vi "uTTA_CutCoolingToSection.vi"(4 "uTTA_MetaData":T1={"Tsamp,fast"=1.25, "Tsamp,slow"=20480.0, "Samples/Decade"=200, "Max.Divider"=14, "T_Preheat"=60.0, "T_Heat"=2400.0, "T_Cool"=10800.0, "Cooling Start Block"=601, " Total Blocks"=3250, "SuspectLines"=[], "Cool Voltage"=0.0, "Cool Volt Deviation"=0.0, "Heating Power"=0.0, "Chip Size"=0.0, "Interpolation Offset"=0.0, "Interpolation Factor m"=0.0, "No Suspect Lines"=0} {"No Suspect Lines" format="%.3pV"; "Interpolation Factor m" format="%.2g"; "Interpolation Offset" format="%.2g"; "Chip Size" format="%.2gmm²"; "Heating Power" format="%.3pW"; "Cool Volt Deviation" format="%.3pV"; "Cool Voltage" format="%.3pV"}, 5 "MeasData_in":T2, 6 "Off-Voltage":dbl=0.3 caption="Treshhold" min=-10.0 max=10.0 step=0.01, 7 "Cut at Off-Voltage":bool=TRUE caption="Enable") -> (0 "uTTA_MetaData_out":T1 {"No Suspect Lines" format="%.3pV"; "Interpolation Factor m" format="%.2g"; "Interpolation Offset" format="%.2g"; "Chip Size" format="%.2gmm²"; "Heating Power" format="%.3pW"; "Cool Volt Deviation" format="%.3pV"; "Cool Voltage" format="%.3pV"; "Tsamp,fast" format="%#_3gus"; "Tsamp,slow" format="%#_3gus"; "T_Preheat" format="%#_3gs"; "T_Heat" format="%#_3gs"; "T_Cool" format="%#_3gs"}, 1 "MeasData_out":T2, 2 "Index":i32, 3 "Graph_out":cluster{"Array":dbl[], "Array":dbl[]}[](array[cluster]))   [LabVIEW 2021]
uses:
  CTL_uTTA_MeasurementData.ctl
  uTTA_MetaData.ctl
  <vilib>/Analysis/NI_AALBase.lvlib
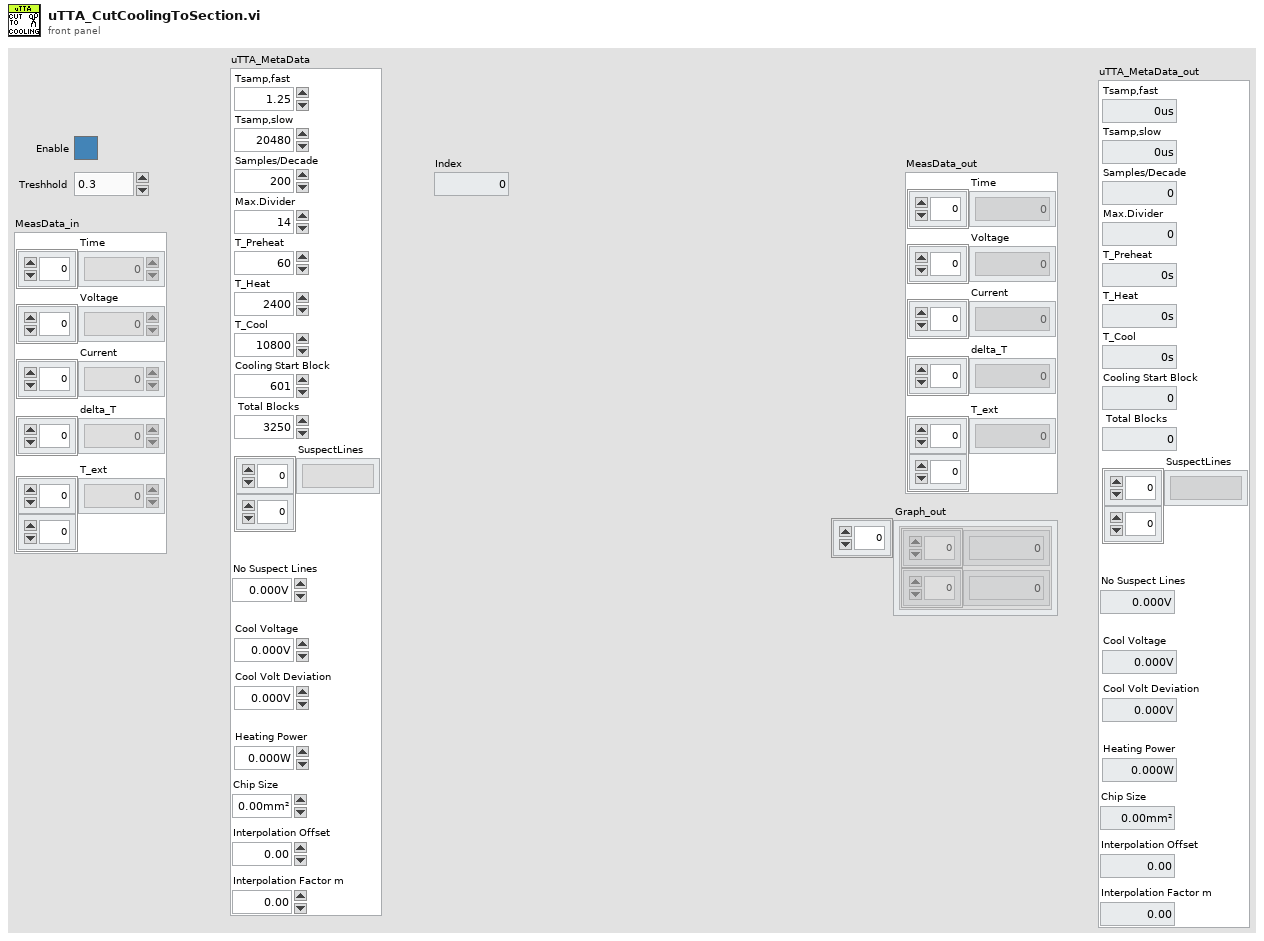
[diagram p1: front panel]
types:
  T1 = typedef "uTTA_MetaData.ctl" = cluster{"Tsamp,fast":dbl, "Tsamp,slow":dbl, "Samples/Decade":u32, "Max.Divider":u32, "T_Preheat":dbl, "T_Heat":dbl, "T_Cool":dbl, "Cooling Start Block":u32, " Total Blocks":u32, "SuspectLines":string[][], "Cool Voltage":dbl, "Cool Volt Deviation":dbl, "Heating Power":dbl, "Chip Size":dbl, "Interpolation Offset":dbl, "Interpolation Factor m":dbl, "No Suspect Lines":u32}
  T2 = typedef "CTL_uTTA_MeasurementData.ctl" = cluster{"Time":dbl[], "Voltage":dbl[], "Current":dbl[], "delta_T":dbl[], "T_ext":dbl[][]}
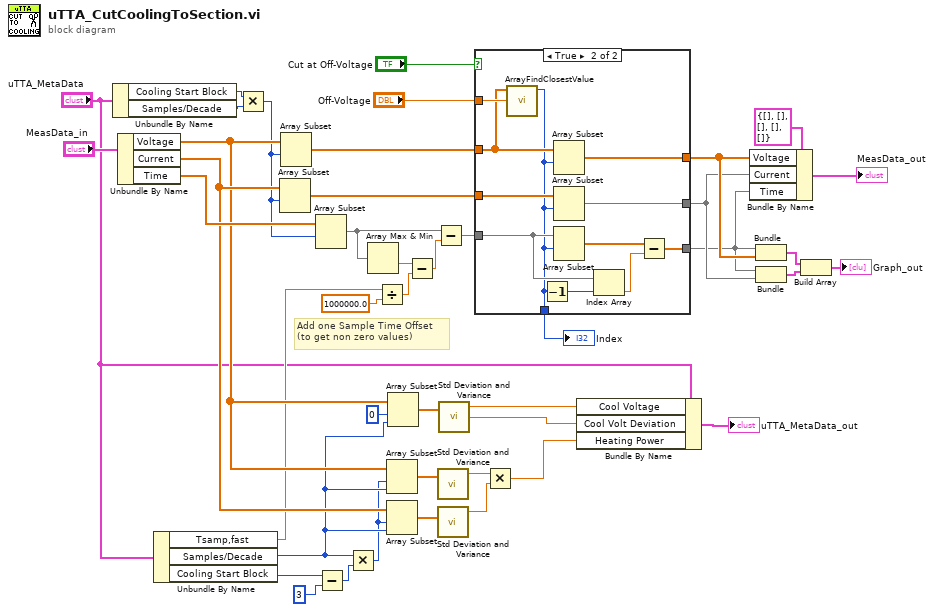
[diagram p0: block diagram]
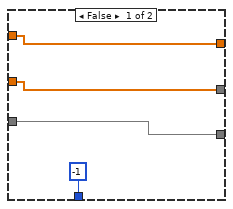
[diagram p2: hidden frame]
diagram:
  # "Add one Sample Time Offset\n(to get non zero values)"
  n1 = Unbundle By Name("uTTA_MetaData") -> ("Cooling Start Block"=w30:u32, "Samples/Decade"=w31:u32)
  n2 = Unbundle By Name("MeasData_in") -> ("Voltage"=w36:dbl[], "Current"=w37:dbl[], "Time"=w38:dbl[])
  n3 = Unbundle By Name("uTTA_MetaData") -> ("Tsamp,fast"=w34:dbl, "Samples/Decade"=w33:u32, "Cooling Start Block"=w32:u32)
  n4 = Multiply(x=w30, y=w31) -> (x*y=w14:u32)
  n5 = Array Subset(array=w37, index=w14) -> (w19:dbl[])  [unwired: 1 in]
  n6 = Array Subset(array=w36, index=w14) -> (w18:dbl[])  [unwired: 1 in]
  n7 = Array Subset(array=w38, index=w14) -> (w17:dbl[])  [unwired: 1 in]
  n8 = Subtract(x=w32, y=u32 3) -> (x-y=w24:u32)
  n9 = Multiply(x=w33, y=w24) -> (x*y=w25:u32)
  n10 = Array Max & Min(array=w17) -> (min value=w15:dbl)  [unwired: 3 out]
  n11 = Divide(x=w34, y=1000000.0) -> (x/y=w11:dbl)
  n12 = Array Subset(array=w36, index=w25, length=w33) -> (w26:dbl[])
  n13 = Array Subset(array=w37, index=w25, length=w33) -> (w27:dbl[])
  n14 = Array Subset(array=w36, index=0, length=w33) -> (w22:dbl[])
  n15 = Subtract(x=w15, y=w11) -> (x-y=w16:dbl)
  n16 = Subtract(x=w17, y=w16) -> (x-y=w20:dbl[])
  n17 = call <vilib>:"Std Deviation and Variance.vi"("X"=w26) -> ("mean"=w28:dbl)  [unwired: 1 in, 2 out]
  n18 = call <vilib>:"Std Deviation and Variance.vi"("X"=w27) -> ("mean"=w29:dbl)  [unwired: 1 in, 2 out]
  n19 = call <vilib>:"Std Deviation and Variance.vi"("X"=w22) -> ("mean"=w3:dbl, "standard deviation"=w4:dbl)  [unwired: 1 in, 1 out]
  n20 = case shown="True" "Cut at Off-Voltage" {
    tunnel: "Off-Voltage" -> [_ w58]
    tunnel: w18 -> [w47 w57]
    tunnel: [w47 w56] -> w42
    tunnel: w19 -> [w46 w55]
    tunnel: [w46 w54] -> w41
    tunnel: w20 -> [w45 w53]
    tunnel: [w45 w49] -> w40
    tunnel: [-1 ("Index") w48] -> w6
    frame False {
    }
    frame True {
      n21 = call "ArrayFindClosestValue.vi"("Search Item"=w58, "Array"=w57) -> ("Index"=w48:i32)  [unwired: 9 in]
      n22 = Decrement(x=w48) -> (x-1=w52:i32)
      n23 = Array Subset(array=w57, index=w48) -> (w56:dbl[])  [unwired: 1 in]
      n24 = Array Subset(array=w55, index=w48) -> (w54:dbl[])  [unwired: 1 in]
      n25 = Array Subset(array=w53, index=w48) -> (w50:dbl[])  [unwired: 1 in]
      n26 = Index Array(array=w53, index=w52) -> (element=w51:dbl)
      n27 = Subtract(x=w50, y=w51) -> (x-y=w49:dbl[])
    }
  }
  "Index" <- w6
  n28 = Multiply(x=w28, y=w29) -> (x*y=w5:dbl)
  n29 = Bundle By Name(cluster="uTTA_MetaData", "Cool Voltage"=w3, "Cool Volt Deviation"=w4, "Heating Power"=w5) -> (→"uTTA_MetaData_out":T1)
  n30 = Bundle By Name(cluster=T2 {"Time"=[], "Voltage"=[], "Current"=[], "delta_T"=[], "T_ext"=[]} ("MeasData_out"), "Voltage"=w42, "Current"=w41, "Time"=w40) -> (→"MeasData_out":T2)
  n31 = Bundle(w40, w42) -> (w13:cluster{dbl[], dbl[]})  [unwired: 1 in]
  n32 = Bundle(w40, w41) -> (w12:cluster{dbl[], dbl[]})  [unwired: 1 in]
  n33 = Build Array(w13, w12) -> (→"Graph_out":cluster{dbl[], dbl[]}[])
